vi "Initialize RFSA.vi"(5 "N/block":i64, 7 "Reference Level":dbl, 8 "error in (no error)":errorcluster, 9 "IQ Rate":dbl, 10 "Carrier Frequency":dbl, 11 "RFSA Reference In":refnum<k15>) -> (0 "error out":errorcluster, 3 "RFSA Reference Out":refnum<k15>)   [LabVIEW 2021]
uses:
  <instrlib>/niRFSA/niRFSA.llb/niRFSA Configure Spectrum Frequency Center Span.vi
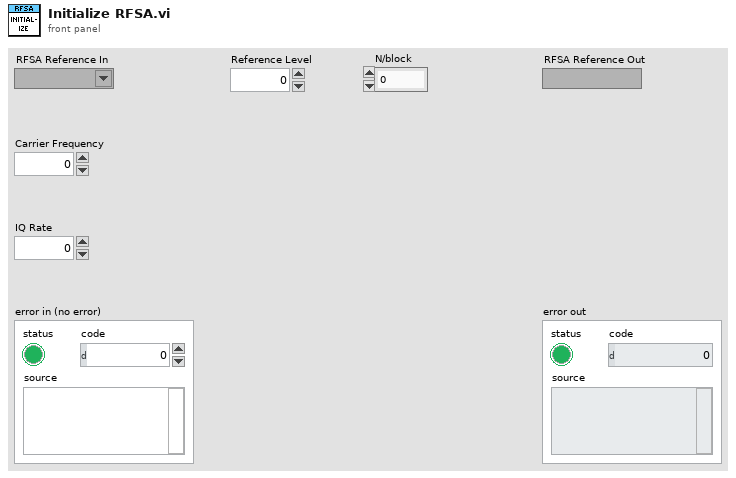
[diagram p1: front panel]
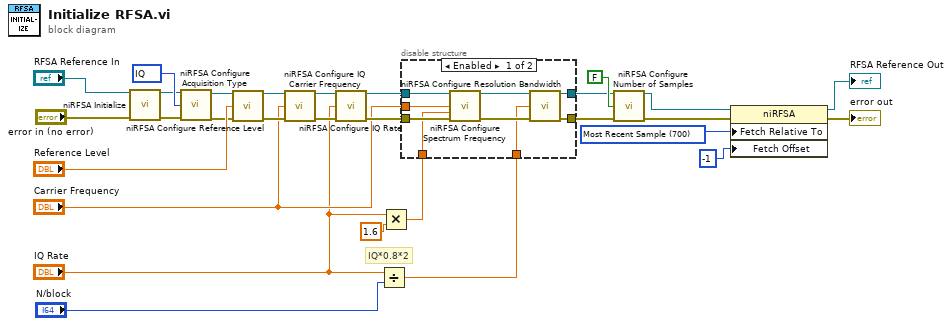
[diagram p0: block diagram]
diagram:
  w24 = 700 items=["Most Recent Sample"=700, "First Sample"=701, "Reference Trigger"=702, "First Pretrigger Sample"=703, "Current Read Position"=704] ("Acquisition:Fetch:Fetch Relative To")
  w20 = 100 items=["IQ"=100, "Spectrum"=101] ("Acquisition:Acquisition Type")
  # "IQ*0.8*2"
  n1 = call <instrlib>:"niRFSA Initialize.vi"("resource name"="RFSA Reference In", "error in"="error in (no error)") -> ("instrument handle out"=w15:refnum<k15>, "error out"=w14:errorcluster)  [unwired: 12 in]
  n2 = call <instrlib>:"niRFSA Configure Acquisition Type.vi"("instrument handle"=w15, "acquisition type"=w20, "error in"=w14) -> ("instrument handle out"=w12:refnum<k15>, "error out"=w13:errorcluster)  [unwired: 11 in]
  n3 = call <instrlib>:"niRFSA Configure Reference Level.vi"("instrument handle"=w12, "reference level (dBm)"="Reference Level", "error in"=w13) -> ("instrument handle out"=w16:refnum<k15>, "error out"=w17:errorcluster)  [unwired: 11 in]
  n4 = call <instrlib>:"niRFSA Configure IQ Carrier Frequency.vi"("instrument handle"=w16, "carrier frequency"="Carrier Frequency", "error in"=w17) -> ("instrument handle out"=w18:refnum<k15>, "error out"=w19:errorcluster)  [unwired: 11 in]
  n5 = call <instrlib>:"niRFSA Configure IQ Rate.vi"("instrument handle"=w18, "IQ rate (S/s)"="IQ Rate", "error in"=w19) -> ("instrument handle out"=w9:refnum<k15>, "error out"=w10:errorcluster)  [unwired: 11 in]
  n6 = Divide(x="IQ Rate", y="N/block") -> (x/y=w1:dbl)
  n7 = Multiply(x="IQ Rate", y=1.6) -> (x*y=w6:dbl)
  n8 = disable-structure shown="Enabled" {
    disable-tunnel: w10 -> [w38 w39]
    disable-tunnel: w9 -> [w37 w40]
    disable-tunnel: "Carrier Frequency" -> [w36 _]
    disable-tunnel: w6 -> [w35 _]
    disable-tunnel: [w33 w39] -> w5
    disable-tunnel: [w31 w40] -> w4
    disable-tunnel: w1 -> [w30 _]
    frame Enabled {
      n9 = call-poly <instrlib>:"niRFSA Configure Spectrum Frequency.vi"("instrument handle"=w37, "frequency"=w36, "span"=w35, "error in"=w38) -> ("instrument handle out"=w32:refnum<k15>, "error out"=w34:errorcluster)  [unwired: 10 in]
      n10 = call <instrlib>:"niRFSA Configure Resolution Bandwidth.vi"("instrument handle"=w32, "resolution bandwidth (Hz)"=w30, "error in"=w34) -> ("instrument handle out"=w31:refnum<k15>, "error out"=w33:errorcluster)  [unwired: 11 in]
    }
    frame Disabled {
    }
  }
  n11 = call <instrlib>:"niRFSA Configure Number of Samples.vi"("instrument handle"=w4, "number of samples is finite"=FALSE, "error in"=w5) -> ("instrument handle out"=w27:refnum<k15>, "error out"=w25:errorcluster)  [unwired: 11 in]
  n12 = property class="niRFSA"(reference=w27, error in=w25, "Fetch Relative To"=w24, "Fetch Offset"=i64 -1 ("Acquisition:Fetch:Fetch Offset")) -> (reference out=→"RFSA Reference Out":refnum<k15>, error out=→"error out":errorcluster)
